vi "quiz 2 2021-2 maquina de estados.vi"() -> ()   [LabVIEW 2020]
panel:
  in  "inicio":bool
  in  "reset":bool
  in  "stop":bool
  out "devuelta":dbl
  out "coins":dbl
  out "String":string
  in  "candies":bool
  in  "cool drink":bool
  in  "coffee":bool
  in  "snacks":bool
  in  "20":bool
  in  "10":bool
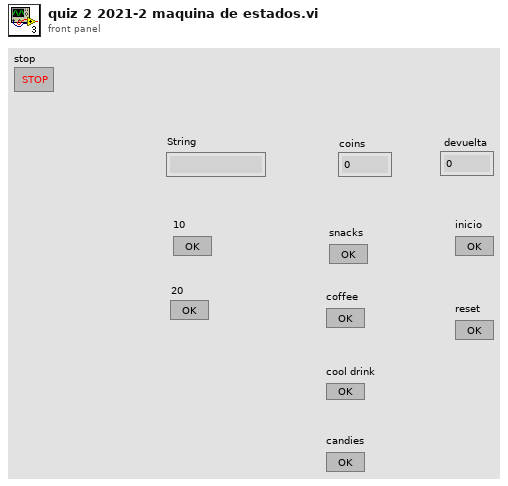
[diagram p1: front panel]
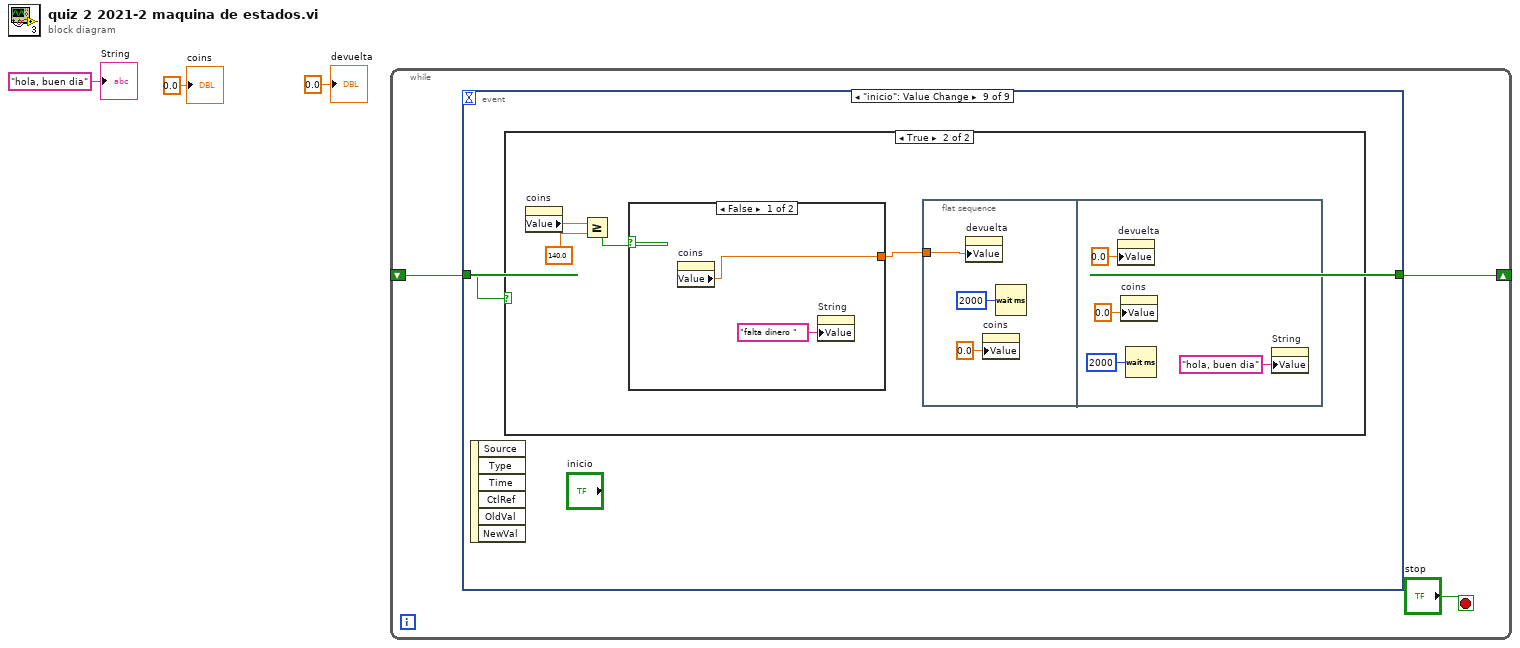
[diagram p0: block diagram]
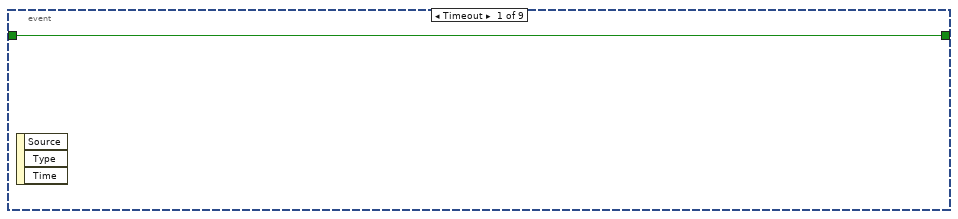
[diagram p2: hidden frame]
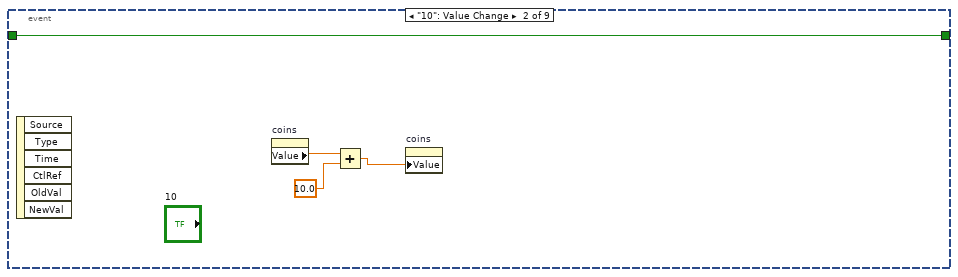
[diagram p3: hidden frame]
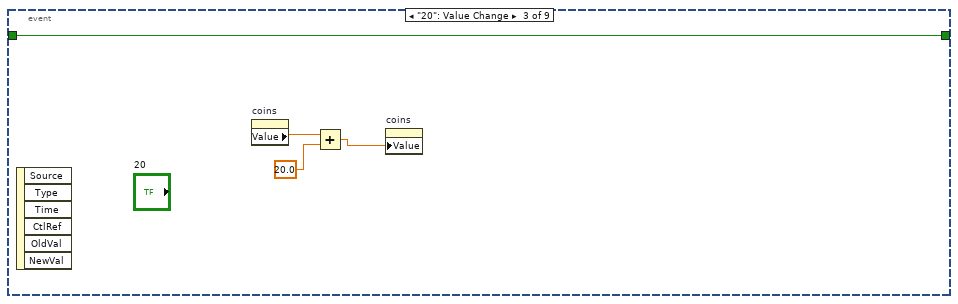
[diagram p4: hidden frame]
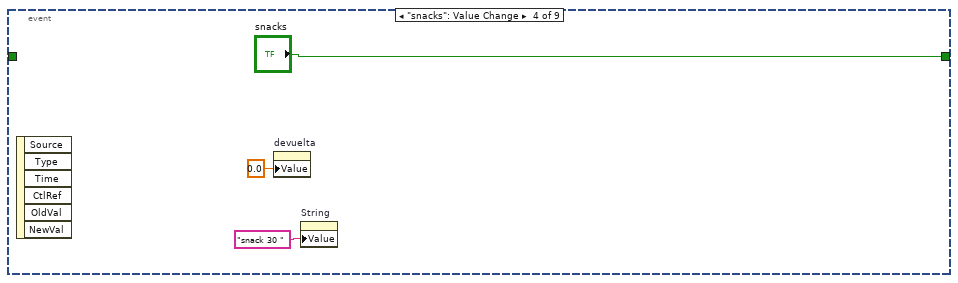
[diagram p5: hidden frame]
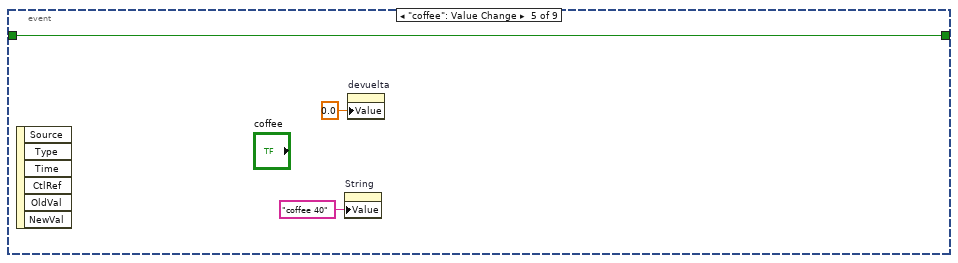
[diagram p6: hidden frame]
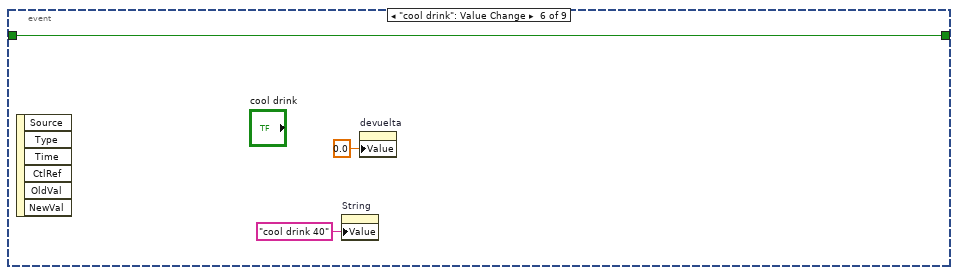
[diagram p7: hidden frame]
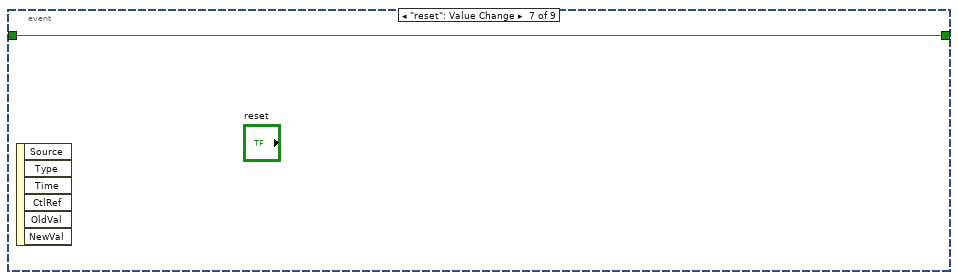
[diagram p8: hidden frame]
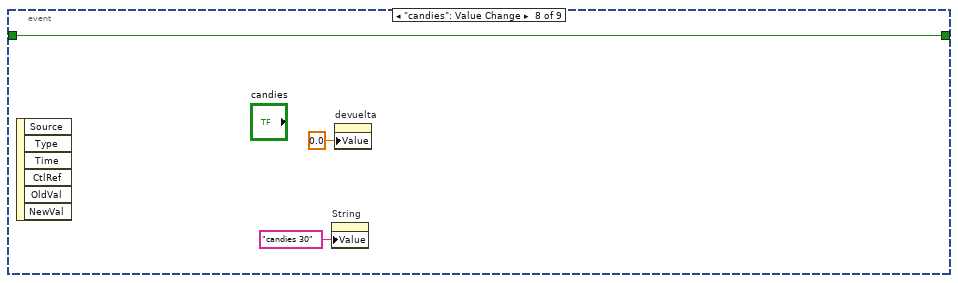
[diagram p9: hidden frame]
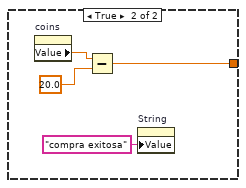
[diagram p11: hidden frame]
diagram:
  n1 = while {
    shift-right: [w5] -> _
    shift-left: _ -> [w4]
    stop <- "stop" stop-if-true
    n2 = event shown="[8] \"inicio\": Value Change" {
      selector: _ -> [_ _ _ _ _ _ _ _ _]
      dyn-events: _ -> [_ _ _ _ _ _ _ _ _]
      timeout: _ -> [_ _ _ _ _ _ _ _ _]
      tunnel: [w7 w8 w12 "snacks" w19 w22 w25 w26 _] -> w5
      tunnel: w4 -> [w7 w8 w12 _ w19 w22 w25 w26 w29]
      event Timeout {
        n3 = event-data() -> ()  [unwired: 1 in, 3 out]
      }
      event "10": Value Change {
        n4 = event-data() -> ()  [unwired: 1 in, 6 out]
        n5 = property on="coins" class="DigNum (strict)"() -> ("Value"=w11:dbl)  [unwired: 2 in, 2 out]
        n6 = Add(x=w11, y=10.0) -> (x+y=w10:dbl)
        n7 = property on="coins" class="DigNum (strict)"("Value"=w10) -> ()  [unwired: 2 in, 2 out]
      }
      event "20": Value Change {
        n8 = event-data() -> ()  [unwired: 1 in, 6 out]
        n9 = property on="coins" class="DigNum (strict)"() -> ("Value"=w15:dbl)  [unwired: 2 in, 2 out]
        n10 = Add(x=w15, y=20.0) -> (x+y=w14:dbl)
        n11 = property on="coins" class="DigNum (strict)"("Value"=w14) -> ()  [unwired: 2 in, 2 out]
      }
      event "snacks": Value Change {
        n12 = event-data() -> ()  [unwired: 1 in, 6 out]
        n13 = property on="devuelta" class="DigNum (strict)"("Value"=0.0 ("devuelta")) -> ()  [unwired: 2 in, 2 out]
        n14 = property on="String" class="Str"("Value"="snack 30 " ("String")) -> ()  [unwired: 2 in, 2 out]
      }
      event "coffee": Value Change {
        n15 = event-data() -> ()  [unwired: 1 in, 6 out]
        n16 = property on="String" class="Str"("Value"="coffee 40" ("String")) -> ()  [unwired: 2 in, 2 out]
        n17 = property on="devuelta" class="DigNum (strict)"("Value"=0.0 ("devuelta")) -> ()  [unwired: 2 in, 2 out]
      }
      event "cool drink": Value Change {
        n18 = event-data() -> ()  [unwired: 1 in, 6 out]
        n19 = property on="String" class="Str"("Value"="cool drink 40" ("String")) -> ()  [unwired: 2 in, 2 out]
        n20 = property on="devuelta" class="DigNum (strict)"("Value"=0.0 ("devuelta")) -> ()  [unwired: 2 in, 2 out]
      }
      event "reset": Value Change {
        n21 = event-data() -> ()  [unwired: 1 in, 6 out]
      }
      event "candies": Value Change {
        n22 = event-data() -> ()  [unwired: 1 in, 6 out]
        n23 = property on="String" class="Str"("Value"="candies 30" ("String")) -> ()  [unwired: 2 in, 2 out]
        n24 = property on="devuelta" class="DigNum (strict)"("Value"=0.0 ("devuelta")) -> ()  [unwired: 2 in, 2 out]
      }
      event "inicio": Value Change {
        n25 = event-data() -> ()  [unwired: 1 in, 6 out]
        n26 = case shown="True" w29 {
          frame False {
          }
          frame True {
            n27 = property on="coins" class="DigNum (strict)"() -> ("Value"=w33:dbl)  [unwired: 2 in, 2 out]
            n28 = Greater Or Equal?(x=w33, y=140.0) -> (x >= y?=w31:bool)
            n29 = case shown="False" w31 {
              tunnel: [w41 w43] -> w30
              frame False {
                n30 = property on="coins" class="DigNum (strict)"() -> ("Value"=w41:dbl)  [unwired: 2 in, 2 out]
                n31 = property on="String" class="Str"("Value"="falta dinero " ("String")) -> ()  [unwired: 2 in, 2 out]
              }
              frame True {
                n32 = property on="coins" class="DigNum (strict)"() -> ("Value"=w46:dbl)  [unwired: 2 in, 2 out]
                n33 = Subtract(x=w46, y=20.0) -> (x-y=w43:dbl)
                n34 = property on="String" class="Str"("Value"="compra exitosa" ("String")) -> ()  [unwired: 2 in, 2 out]
              }
            }
            n35 = flat-sequence {
              tunnel: w30 -> [w36]
              frame #0 {
                n36 = property on="devuelta" class="DigNum (strict)"("Value"=w36) -> ()  [unwired: 2 in, 2 out]
                n37 = property on="coins" class="DigNum (strict)"("Value"=0.0 ("coins")) -> ()  [unwired: 2 in, 2 out]
                n38 = Wait (ms)(milliseconds to wait=u32 2000) -> ()  [unwired: 1 out]
              }
              frame #1 {
                n39 = property on="devuelta" class="DigNum (strict)"("Value"=0.0 ("devuelta")) -> ()  [unwired: 2 in, 2 out]
                n40 = property on="coins" class="DigNum (strict)"("Value"=0.0 ("coins")) -> ()  [unwired: 2 in, 2 out]
                n41 = Wait (ms)(milliseconds to wait=u32 2000) -> ()  [unwired: 1 out]
                n42 = property on="String" class="Str"("Value"="hola, buen dia" ("String")) -> ()  [unwired: 2 in, 2 out]
              }
            }
          }
        }
      }
    }
  }
  "String" <- "hola, buen dia" ("String")
  "coins" <- 0.0 ("coins")
  "devuelta" <- 0.0 ("devuelta")
